vi "Set Index.vi"(8 "error in":errorcluster, 10 "Index":u16 format="%04x", 11 "PDO Communication Parameter in":refnum<class "PDO Communication Parameter.lvclass">) -> (0 "error out":errorcluster, 3 "PDO Communication Parameter out":refnum<class "PDO Communication Parameter.lvclass">)   [LabVIEW 2020, in "CANopen.lvlib" / "PDO Communication Parameter.lvclass"]
uses:
  PDO Communication Parameter.lvclass
  PDO Communication Parameter.lvclass/PDO Communication Parameter.ctl
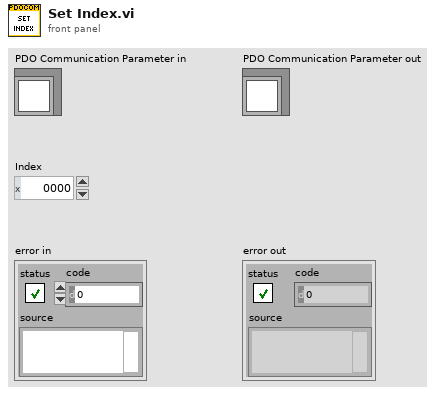
[diagram p1: front panel]
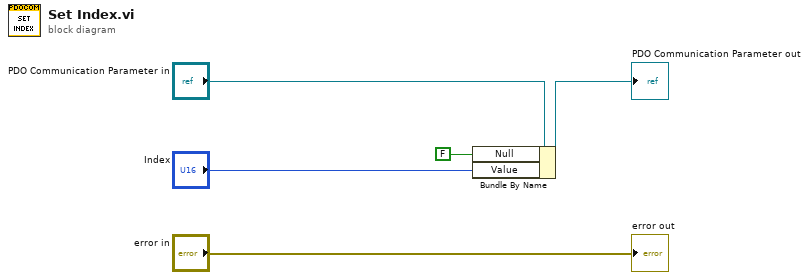
[diagram p0: block diagram]
diagram:
  n1 = Bundle By Name(cluster="PDO Communication Parameter in", "Null"=FALSE ("Index.Null"), "Value"="Index") -> (→"PDO Communication Parameter out":refnum<class "PDO Communication Parameter.lvclass">)
  "error out" <- "error in"
